vi "ConcatenateIfPresent.vi"(5 "prependString":string, 9 "appendString":string) -> (8 "outputString":string)   [LabVIEW 2016]
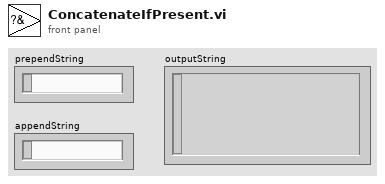
[diagram p1: front panel]
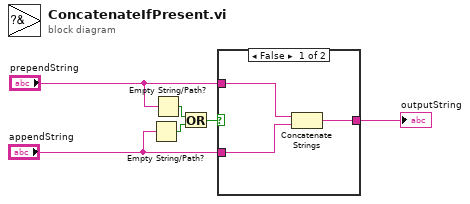
[diagram p0: block diagram]
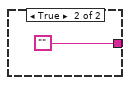
[diagram p2: hidden frame]
diagram:
  n1 = Empty String/Path?(string/path="appendString") -> (empty?=w3:bool)
  n2 = Empty String/Path?(string/path="prependString") -> (empty?=w2:bool)
  n3 = Or(x=w2, y=w3) -> (x .or. y?=w1:bool)
  n4 = case shown="False" w1 {
    tunnel: "appendString" -> [w7 _]
    tunnel: [w9 ""] -> w5
    tunnel: "prependString" -> [w8 _]
    frame False {
      n5 = Concatenate Strings(w8, w7) -> (w9:string)
    }
    frame True {
    }
  }
  "outputString" <- w5
